vi "buffer to data array.vi"(8 "set para 2":T1, 10 "buffer":u16[](array[numeric]), 11 "i":i32) -> (2 "data":dbl[](array[numeric]))   [LabVIEW 2011]
panel:
  out "set para 3":T1
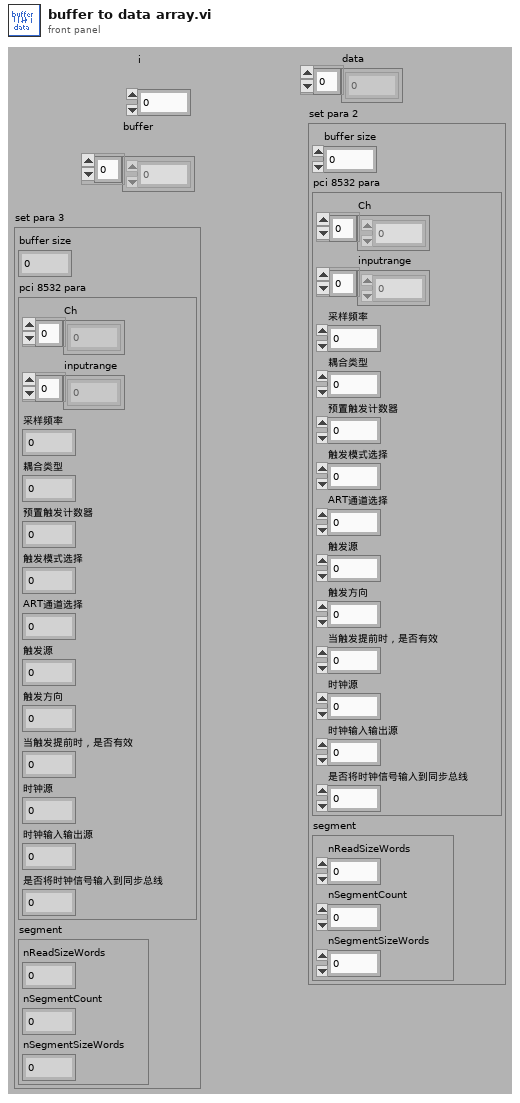
[diagram p1: front panel]
types:
  T1 = cluster{"buffer size":i32, "pci 8532 para":cluster{"Ch":i32[], "inputrange":i32[], "采样频率":i32, "耦合类型":i32, "预置触发计数器":i32, "触发模式选择":i32, "ART通道选择":i32, "触发源":i32, "触发方向":i32, "当触发提前时，是否有效":i32, "时钟源":i32, "时钟输入输出源":i32, "是否将时钟信号输入到同步总线":i32}, "segment":cluster{"nReadSizeWords":i32, "nSegmentCount":i32, "nSegmentSizeWords":i32}}
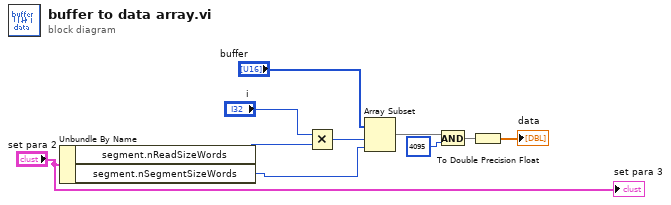
[diagram p0: block diagram]
diagram:
  n1 = Unbundle By Name("set para 2") -> ("segment.nReadSizeWords"=w2:i32, "segment.nSegmentSizeWords"=w1:i32)
  n2 = Multiply(x="i", y=w2) -> (x*y=w10:i32)
  n3 = Array Subset(array="buffer", index=w10, length=w1) -> (w7:u16[])
  n4 = And(x=w7, y=u16 4095) -> (x .and. y?=w8:u16[])
  n5 = To Double Precision Float(number=w8) -> (double precision float=→"data":dbl[])
  "set para 3" <- "set para 2"
